vi "createDisabledList.vi"(8 "error in (no error)":errorcluster, 11 "ILCCommunications in":refnum<class "ILCCommunications.lvclass">) -> (0 "error out":errorcluster, 3 "ILCCommunications out":refnum<class "ILCCommunications.lvclass">)   [LabVIEW 2016, in "ILCCommunications.lvclass"]
uses:
  ILCCommunications.lvclass
  Common_RT_Modbus/ModbusBuffer/ModbusBuffer.lvclass
  Common_RT_Modbus/ModbusBuffer/ModbusBuffer.lvclass/ModbusBuffer.ctl
  ILCCommunications.lvclass/ILCCommunications.ctl
  Common_RT_FAILC/FAILC/FAILC.lvclass/FAILC.ctl
  Common_RT_HPILC/HPILC/HPILC.lvclass/HPILC.ctl
  Common_RT_ILC/ILC/ILC.lvclass/ILC.ctl
  Common_RT_Modbus/ModbusBuffer/writeSoftwareTrigger.vi
  Common_RT_Modbus/ModbusBuffer/writeHeader.vi
  Common_RT_FAILC/FAILC/addBroadcastFreezeSensorValuesFrame.vi
  Common_RT_HPILC/HPILC/addBroadcastFreezeSensorValuesFrame.vi
  Common_RT_Modbus/ModbusBuffer/writeTimestamp.vi
  reportFAForceAndStatus.vi
  reportHPForceAndStatus.vi
  reportHPServerStatus.vi
  Common_RT_Modbus/ModbusBuffer/writeTriggerIRQ.vi
  Common_RT_Modbus/ModbusBuffer/writeU8.vi
  Common_RT_Modbus/ModbusBuffer/writeCRC.vi
  Common_RT_Modbus/ModbusBuffer/writeEndOfFrame.vi
  Common_RT_Modbus/ModbusBuffer/writeDelay.vi
  Common_RT_FAILC/FAILC/addForceAndStatusFrame.vi
  Common_RT_HPILC/HPILC/createForceAndStatusFrame.vi
  reportServerStatus.vi
  Common_RT_Modbus/ModbusBuffer/writeByteInstruction.vi
  Common_RT_Modbus/ModbusBuffer/calculateCRC.vi
  Common_RT_ILC/ILC/getILCData.vi
  Common_RT_Modbus/ModbusBuffer/writeWaitForRx.vi
  Common_RT_ILC/ILC/addReportServerStatusFrame.vi
  Common_RT_FAILC/FAILC/FAILC.lvclass
  D:/Code/ts_M1M3Support/Common_RT_ILC/ILC/ILC.lvclass
  Common_RT_HPILC/HPILC/HPILC.lvclass
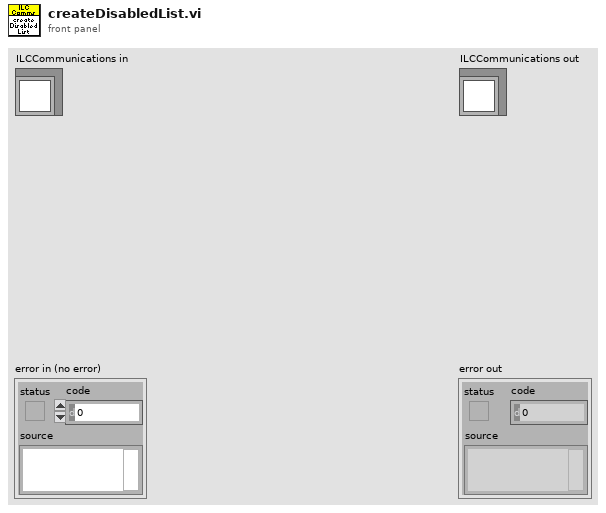
[diagram p1: front panel]
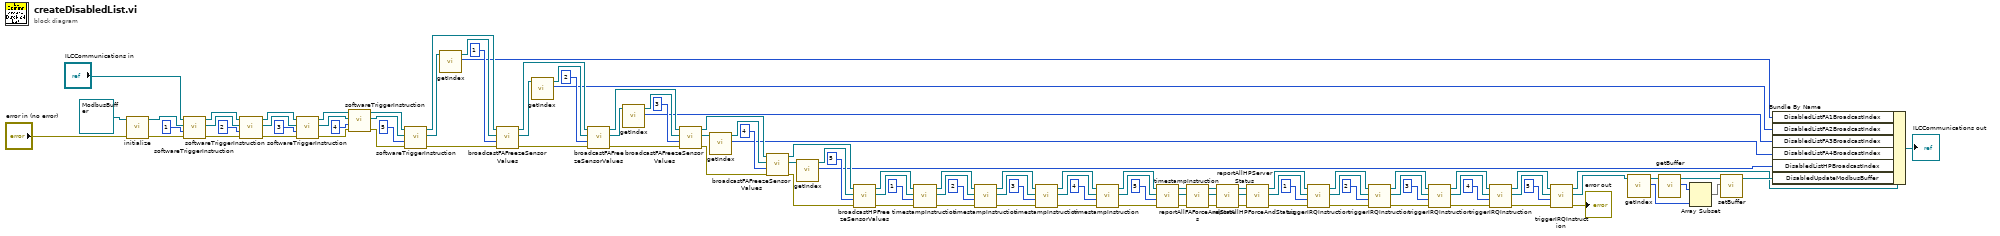
[diagram p0: block diagram]
diagram:
  n1 = call "initialize.vi"("error in (no error)"="error in (no error)", "ModbusBuffer in"=refnum<class "ModbusBuffer.lvclass"> refnum ("RTModbus.lvlib:ModbusBuffer.lvclass")) -> ("error out"=w82:errorcluster, "ModbusBuffer out"=w87:refnum<class "ModbusBuffer.lvclass">)  [unwired: 8 in]
  n2 = call "softwareTriggerInstruction.vi"("error in (no error)"=w82, "Subnet"=u8 1, "ModbusBuffer in"=w87, "ILCCommunications in"="ILCCommunications in") -> ("error out"=w81:errorcluster, "ModbusBuffer out"=w86:refnum<class "ModbusBuffer.lvclass">, "ILCCommunications out"=w91:refnum<class "ILCCommunications.lvclass">)  [unwired: 5 in]
  n3 = call "softwareTriggerInstruction.vi"("error in (no error)"=w81, "Subnet"=u8 2, "ModbusBuffer in"=w86, "ILCCommunications in"=w91) -> ("error out"=w80:errorcluster, "ModbusBuffer out"=w85:refnum<class "ModbusBuffer.lvclass">, "ILCCommunications out"=w90:refnum<class "ILCCommunications.lvclass">)  [unwired: 5 in]
  n4 = call "softwareTriggerInstruction.vi"("error in (no error)"=w80, "Subnet"=u8 3, "ModbusBuffer in"=w85, "ILCCommunications in"=w90) -> ("error out"=w79:errorcluster, "ModbusBuffer out"=w84:refnum<class "ModbusBuffer.lvclass">, "ILCCommunications out"=w89:refnum<class "ILCCommunications.lvclass">)  [unwired: 5 in]
  n5 = call "softwareTriggerInstruction.vi"("error in (no error)"=w79, "Subnet"=u8 4, "ModbusBuffer in"=w84, "ILCCommunications in"=w89) -> ("error out"=w78:errorcluster, "ModbusBuffer out"=w83:refnum<class "ModbusBuffer.lvclass">, "ILCCommunications out"=w88:refnum<class "ILCCommunications.lvclass">)  [unwired: 5 in]
  n6 = call "softwareTriggerInstruction.vi"("error in (no error)"=w78, "Subnet"=u8 5, "ModbusBuffer in"=w83, "ILCCommunications in"=w88) -> ("error out"=w44:errorcluster, "ModbusBuffer out"=w93:refnum<class "ModbusBuffer.lvclass">, "ILCCommunications out"=w57:refnum<class "ILCCommunications.lvclass">)  [unwired: 5 in]
  n7 = call "getIndex.vi"("ModbusBuffer in"=w93) -> ("Index"=w24:i32, "ModbusBuffer out"=w53:refnum<class "ModbusBuffer.lvclass">)  [unwired: 9 in]
  n8 = call "broadcastFAFreezeSensorValues.vi"("error in (no error)"=w44, "Subnet"=u8 1, "ModbusBuffer in"=w53, "ILCCommunications in"=w57) -> ("error out"=w43:errorcluster, "ModbusBuffer out"=w52:refnum<class "ModbusBuffer.lvclass">, "ILCCommunications out"=w56:refnum<class "ILCCommunications.lvclass">)  [unwired: 5 in]
  n9 = call "getIndex.vi"("ModbusBuffer in"=w52) -> ("Index"=w23:i32, "ModbusBuffer out"=w51:refnum<class "ModbusBuffer.lvclass">)  [unwired: 9 in]
  n10 = call "broadcastFAFreezeSensorValues.vi"("error in (no error)"=w43, "Subnet"=u8 2, "ModbusBuffer in"=w51, "ILCCommunications in"=w56) -> ("error out"=w42:errorcluster, "ModbusBuffer out"=w50:refnum<class "ModbusBuffer.lvclass">, "ILCCommunications out"=w55:refnum<class "ILCCommunications.lvclass">)  [unwired: 5 in]
  n11 = call "getIndex.vi"("ModbusBuffer in"=w50) -> ("Index"=w22:i32, "ModbusBuffer out"=w49:refnum<class "ModbusBuffer.lvclass">)  [unwired: 9 in]
  n12 = call "broadcastFAFreezeSensorValues.vi"("error in (no error)"=w42, "Subnet"=u8 3, "ModbusBuffer in"=w49, "ILCCommunications in"=w55) -> ("error out"=w41:errorcluster, "ModbusBuffer out"=w48:refnum<class "ModbusBuffer.lvclass">, "ILCCommunications out"=w54:refnum<class "ILCCommunications.lvclass">)  [unwired: 5 in]
  n13 = call "getIndex.vi"("ModbusBuffer in"=w48) -> ("Index"=w21:i32, "ModbusBuffer out"=w47:refnum<class "ModbusBuffer.lvclass">)  [unwired: 9 in]
  n14 = call "broadcastFAFreezeSensorValues.vi"("error in (no error)"=w41, "Subnet"=u8 4, "ModbusBuffer in"=w47, "ILCCommunications in"=w54) -> ("error out"=w40:errorcluster, "ModbusBuffer out"=w46:refnum<class "ModbusBuffer.lvclass">, "ILCCommunications out"=w38:refnum<class "ILCCommunications.lvclass">)  [unwired: 5 in]
  n15 = call "getIndex.vi"("ModbusBuffer in"=w46) -> ("Index"=w20:i32, "ModbusBuffer out"=w45:refnum<class "ModbusBuffer.lvclass">)  [unwired: 9 in]
  n16 = call "broadcastHPFreezeSensorValues.vi"("error in (no error)"=w40, "Subnet"=u8 5, "ModbusBuffer in"=w45, "ILCCommunications in"=w38) -> ("error out"=w39:errorcluster, "ModbusBuffer out"=w36:refnum<class "ModbusBuffer.lvclass">, "ILCCommunications out"=w37:refnum<class "ILCCommunications.lvclass">)  [unwired: 5 in]
  n17 = call "timestampInstruction.vi"("error in (no error)"=w39, "Subnet"=u8 1, "ModbusBuffer in"=w36, "ILCCommunications in"=w37) -> ("error out"=w65:errorcluster, "ModbusBuffer out"=w69:refnum<class "ModbusBuffer.lvclass">, "ILCCommunications out"=w73:refnum<class "ILCCommunications.lvclass">)  [unwired: 5 in]
  n18 = call "timestampInstruction.vi"("error in (no error)"=w65, "Subnet"=u8 2, "ModbusBuffer in"=w69, "ILCCommunications in"=w73) -> ("error out"=w64:errorcluster, "ModbusBuffer out"=w68:refnum<class "ModbusBuffer.lvclass">, "ILCCommunications out"=w72:refnum<class "ILCCommunications.lvclass">)  [unwired: 5 in]
  n19 = call "timestampInstruction.vi"("error in (no error)"=w64, "Subnet"=u8 3, "ModbusBuffer in"=w68, "ILCCommunications in"=w72) -> ("error out"=w63:errorcluster, "ModbusBuffer out"=w67:refnum<class "ModbusBuffer.lvclass">, "ILCCommunications out"=w71:refnum<class "ILCCommunications.lvclass">)  [unwired: 5 in]
  n20 = call "timestampInstruction.vi"("error in (no error)"=w63, "Subnet"=u8 4, "ModbusBuffer in"=w67, "ILCCommunications in"=w71) -> ("error out"=w62:errorcluster, "ModbusBuffer out"=w66:refnum<class "ModbusBuffer.lvclass">, "ILCCommunications out"=w70:refnum<class "ILCCommunications.lvclass">)  [unwired: 5 in]
  n21 = call "timestampInstruction.vi"("error in (no error)"=w62, "Subnet"=u8 5, "ModbusBuffer in"=w66, "ILCCommunications in"=w70) -> ("error out"=w25:errorcluster, "ModbusBuffer out"=w28:refnum<class "ModbusBuffer.lvclass">, "ILCCommunications out"=w30:refnum<class "ILCCommunications.lvclass">)  [unwired: 5 in]
  n22 = call "reportAllFAForceAndStatus.vi"("error in (no error)"=w25, "ModbusBuffer in"=w28, "ILCCommunications in"=w30) -> ("error out"=w26:errorcluster, "ModbusBuffer out"=w27:refnum<class "ModbusBuffer.lvclass">, "ILCCommunications out"=w29:refnum<class "ILCCommunications.lvclass">)  [unwired: 6 in]
  n23 = call "reportAllHPForceAndStatus.vi"("error in (no error)"=w26, "ModbusBuffer in"=w27, "ILCCommunications in"=w29) -> ("error out"=w104:errorcluster, "ModbusBuffer out"=w110:refnum<class "ModbusBuffer.lvclass">, "ILCCommunications out"=w111:refnum<class "ILCCommunications.lvclass">)  [unwired: 6 in]
  n24 = call "reportAllHPServerStatus.vi"("error in (no error)"=w104, "ModbusBuffer in"=w110, "ILCCommunications in"=w111) -> ("error out"=w9:errorcluster, "ModbusBuffer out"=w14:refnum<class "ModbusBuffer.lvclass">, "ILCCommunications out"=w19:refnum<class "ILCCommunications.lvclass">)  [unwired: 6 in]
  n25 = call "triggerIRQInstruction.vi"("error in (no error)"=w9, "Subnet"=u8 1, "ModbusBuffer in"=w14, "ILCCommunications in"=w19) -> ("error out"=w8:errorcluster, "ModbusBuffer out"=w13:refnum<class "ModbusBuffer.lvclass">, "ILCCommunications out"=w18:refnum<class "ILCCommunications.lvclass">)  [unwired: 5 in]
  n26 = call "triggerIRQInstruction.vi"("error in (no error)"=w8, "Subnet"=u8 2, "ModbusBuffer in"=w13, "ILCCommunications in"=w18) -> ("error out"=w7:errorcluster, "ModbusBuffer out"=w12:refnum<class "ModbusBuffer.lvclass">, "ILCCommunications out"=w17:refnum<class "ILCCommunications.lvclass">)  [unwired: 5 in]
  n27 = call "triggerIRQInstruction.vi"("error in (no error)"=w7, "Subnet"=u8 3, "ModbusBuffer in"=w12, "ILCCommunications in"=w17) -> ("error out"=w6:errorcluster, "ModbusBuffer out"=w11:refnum<class "ModbusBuffer.lvclass">, "ILCCommunications out"=w16:refnum<class "ILCCommunications.lvclass">)  [unwired: 5 in]
  n28 = call "triggerIRQInstruction.vi"("error in (no error)"=w6, "Subnet"=u8 4, "ModbusBuffer in"=w11, "ILCCommunications in"=w16) -> ("error out"=w5:errorcluster, "ModbusBuffer out"=w10:refnum<class "ModbusBuffer.lvclass">, "ILCCommunications out"=w15:refnum<class "ILCCommunications.lvclass">)  [unwired: 5 in]
  n29 = call "triggerIRQInstruction.vi"("error in (no error)"=w5, "Subnet"=u8 5, "ModbusBuffer in"=w10, "ILCCommunications in"=w15) -> ("error out"=→"error out":errorcluster, "ModbusBuffer out"=w98:refnum<class "ModbusBuffer.lvclass">, "ILCCommunications out"=w100:refnum<class "ILCCommunications.lvclass">)  [unwired: 5 in]
  n30 = call "getIndex.vi"("ModbusBuffer in"=w98) -> ("Index"=w108:i32, "ModbusBuffer out"=w107:refnum<class "ModbusBuffer.lvclass">)  [unwired: 9 in]
  n31 = call "getBuffer.vi"("ModbusBuffer in"=w107) -> ("Buffer"=w109:u16[], "ModbusBuffer out"=w105:refnum<class "ModbusBuffer.lvclass">)  [unwired: 9 in]
  n32 = Array Subset(array=w109, length=w108) -> (w106:u16[])  [unwired: 1 in]
  n33 = call "setBuffer.vi"("Buffer"=w106, "ModbusBuffer in"=w105) -> ("ModbusBuffer out"=w102:refnum<class "ModbusBuffer.lvclass">)  [unwired: 9 in]
  n34 = Bundle By Name(cluster=w100, "DisabledListFA1BroadcastIndex"=w24, "DisabledListFA2BroadcastIndex"=w23, "DisabledListFA3BroadcastIndex"=w22, "DisabledListFA4BroadcastIndex"=w21, "DisabledListHPBroadcastIndex"=w20, "DisabledUpdateModbusBuffer"=w102) -> (→"ILCCommunications out":refnum<class "ILCCommunications.lvclass">)
